vi "Parse Data for Logging.vi"(11 "Instrument State":T1) -> (3 "Array":string[](array[string]))   [LabVIEW 2020, in "Omega Platinum Series Plugin.lvlib" / "Logging.lvlib"]
doc: "Parses the Instrument State typedef data into an array of strings to be written to a log file."
uses:
  Logging.lvlib
  Instrument Manager/Instrument State.ctl
  Instrument Manager/Instrument Manager.lvlib
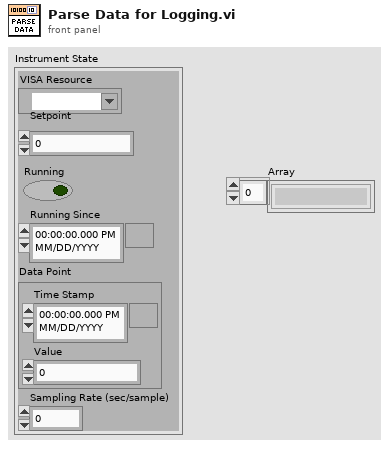
[diagram p1: front panel]
types:
  T1 = typedef "Omega Platinum Series Plugin.lvlib/Instrument Manager.lvlib/Instrument State.ctl" = cluster{"VISA Resource":refnum<visa-resource-name>, "Setpoint":dbl, "Running":bool, "Running Since":timestamp, "Data Point":cluster{"Time Stamp":timestamp, "Value":dbl}, "Sampling Rate (sec/sample)":dbl}
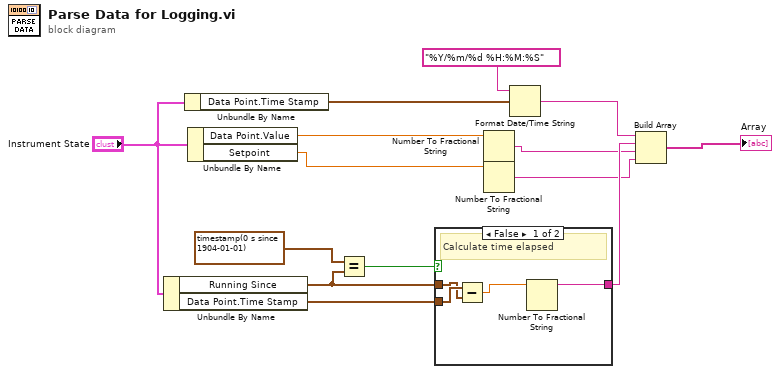
[diagram p0: block diagram]
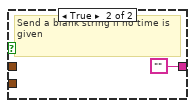
[diagram p2: hidden frame]
diagram:
  n1 = Unbundle By Name("Instrument State") -> ("Running Since"=w5:timestamp, "Data Point.Time Stamp"=w4:timestamp)
  n2 = Unbundle By Name("Instrument State") -> ("Data Point.Time Stamp"=w13:timestamp)
  n3 = Unbundle By Name("Instrument State") -> ("Data Point.Value"=w11:dbl, "Setpoint"=w10:dbl)
  n4 = Equal?(x=timestamp(0 s since 1904-01-01) ("Running Since"), y=w5) -> (x = y?=w7:bool)
  n5 = case shown="False" w7 {
    tunnel: [w15 ""] -> w3
    tunnel: w5 -> [w17 _]
    tunnel: w4 -> [w18 _]
    frame False {
      # "Calculate time elapsed"
      n6 = Subtract(x=w18, y=w17) -> (x-y=w16:dbl)
      n7 = Number To Fractional String(number=w16) -> (F-format string=w15:string)  [unwired: 3 in]
    }
    frame True {
      # "Send a blank string if no time is given"
    }
  }
  n8 = Number To Fractional String(number=w11) -> (F-format string=w2:string)  [unwired: 3 in]
  n9 = Number To Fractional String(number=w10) -> (F-format string=w1:string)  [unwired: 3 in]
  n10 = Format Date/Time String(time format string (%c)="%Y/%m/%d %H:%M:%S", seconds (now)=w13) -> (date/time string=w8:string)  [unwired: 1 in]
  n11 = Build Array(w8, w3, w2, w1) -> (→"Array":string[])
